vi "Find Biggest Outlier.vi"(11 "Line with outlier":T1) -> (2 "Outlier Amount":dbl, 3 "Outlier Index":i32)   [LabVIEW 2017]
uses:
  Vector Library/Line.ctl
  Vector Library/Vector.ctl
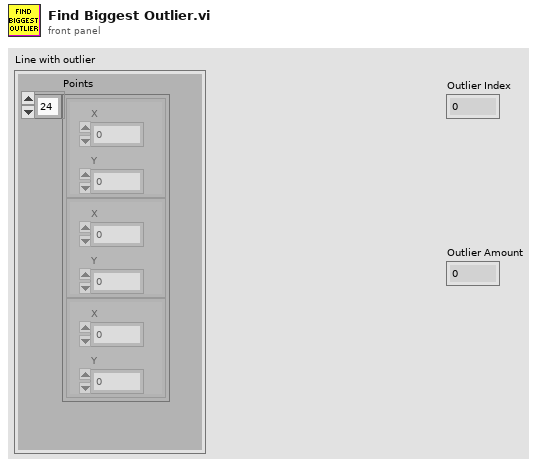
[diagram p1: front panel]
types:
  T1 = typedef "Line.ctl" = cluster{"Points":T2[]}
  T2 = typedef "Vector.ctl" = cluster{"X":dbl, "Y":dbl}
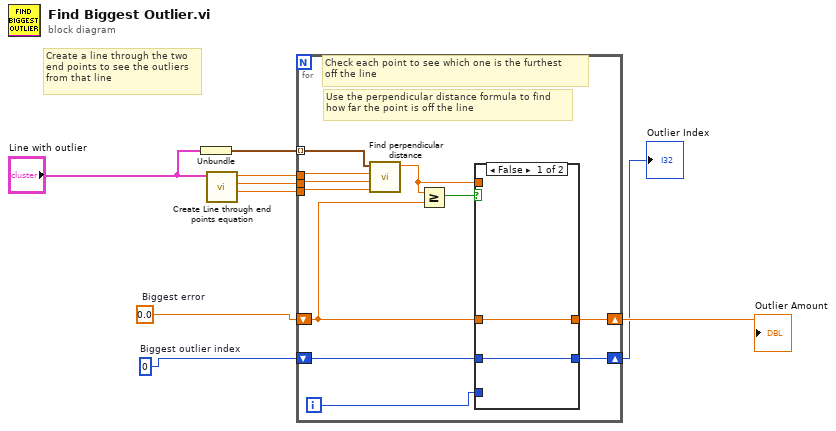
[diagram p0: block diagram]
diagram:
  w8 = 0  # Biggest outlier index
  w9 = 0.0  # Biggest error
  # "Create a line through the two\nend points to see the outliers\nfrom that line"
  n1 = Unbundle("Line with outlier") -> ("Points"=w6:T2[])
  n2 = call "Create Line through end points equation.vi"("Line to create equation for"="Line with outlier") -> ("Y coefficient"=w3:dbl, "X coefficient"=w4:dbl, "Constant"=w5:dbl)  [unwired: 8 in]
  n3 = for {
    shift-right: [w12] -> w2
    shift-left: w9 -> [w15]
    shift-right: [w13] -> w1
    shift-left: w8 -> [w14]
    tunnel: w6 -> [w20] mode=indexing
    tunnel: w5 -> [w19]
    tunnel: w4 -> [w18]
    tunnel: w3 -> [w17]
    i -> [w11]
    # "Use the perpendicular distance formula to find\nhow far the point is off the line"
    # "Check each point to see which one is the furthest \noff the line"
    n4 = call "Find perpendicular distance.vi"("Y coefficient"=w17, "X coefficient"=w18, "Constant"=w19, "Point"=w20) -> ("Distance"=w10:dbl)  [unwired: 7 in]
    n5 = Greater Or Equal?(x=w10, y=w15) -> (x >= y?=w16:bool)
    n6 = case shown="False" w16 {
      tunnel: w15 -> [w21 _]
      tunnel: w14 -> [w22 _]
      tunnel: [w22 w24] -> w13
      tunnel: [w21 w23] -> w12
      tunnel: w11 -> [_ w24]
      tunnel: w10 -> [_ w23]
      frame False {
      }
      frame True {
      }
    }
  }
  "Outlier Index" <- w1
  "Outlier Amount" <- w2
